vi "Read.vi"(8 "error in":errorcluster, 11 "Config File In":path) -> (0 "error out":errorcluster, 2 "ConfigData":T1 {"Inactivity Time" format="%#_g Sec"; "Travel Time" format="%#_g Sec"; "Door Close" format="%#_g Sec"; "Door Open" format="%#_g Sec"}, 3 "Config File Out":path)   [LabVIEW 2020, in "ConfigurationDatabase.lvlib"]
doc: "Reads configuration data from the simulated configuration database.\n[Covers: CD4]"
uses:
  ConfigurationDatabase.lvlib
  Controls/Configuration Data.ctl
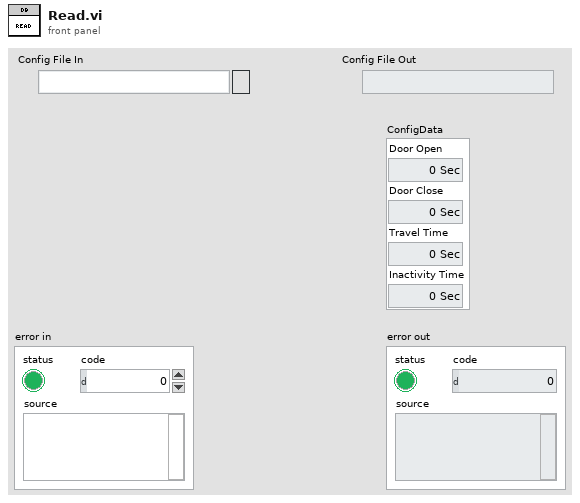
[diagram p1: front panel]
types:
  T1 = typedef "ConfigurationDatabase.lvlib/Configuration Data.ctl" = cluster{"Door Open":dbl, "Door Close":dbl, "Travel Time":dbl, "Inactivity Time":dbl}
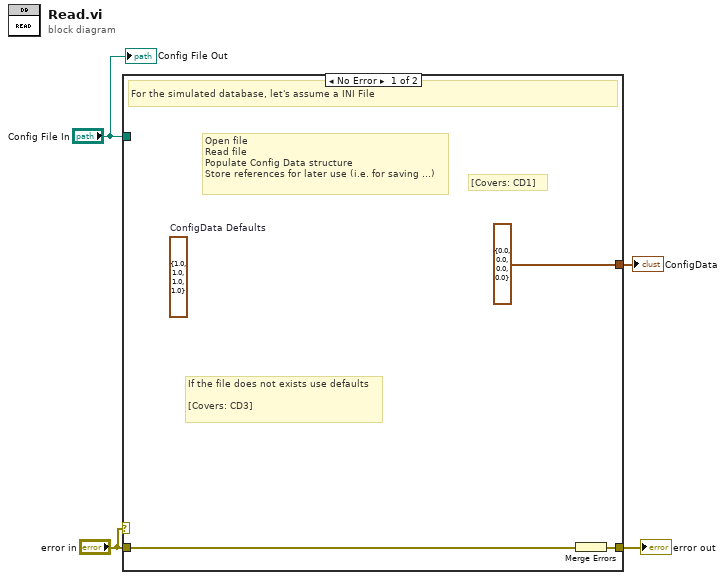
[diagram p0: block diagram]
diagram:
  n1 = case shown="No Error" "error in" {
    tunnel: "error in" -> [w7 w8]
    tunnel: [w6 w8] -> w3
    tunnel: [T1 {"Door Open"=0.0, "Door Close"=0.0, "Travel Time"=0.0, "Inactivity Time"=0.0} ("ConfigData") _] -> w2
    tunnel: "Config File In" -> [_ _]
    frame No Error {
      (unwired) T1 {"Door Open"=1.0, "Door Close"=1.0, "Travel Time"=1.0, "Inactivity Time"=1.0}  # ConfigData Defaults
      # "If the file does not exists use defaults\n\n[Covers: CD3]"
      # "[Covers: CD1]"
      # "Open file\nRead file \nPopulate Config Data structure\nStore references for later use (i.e. for saving ...)"
      # "For the simulated database, let's assume a INI File"
      n2 = Merge Errors(w7) -> (w6:errorcluster)
    }
    frame Error {
    }
  }
  "error out" <- w3
  "ConfigData" <- w2
  "Config File Out" <- "Config File In"
